vi "create.vi"(8 "error in (no error)":errorcluster, 11 "Type":T1=enum."FGEN_NI") -> (0 "error out":errorcluster, 3 "Fgen.lvclass":refnum<class "Arb.lvclass">)   [LabVIEW 2023, in "sweArb.lvlib" / "Arb.lvclass"]
doc: "<b>Author:</b> Wolfgang\n<b>Description:</b> Creates new Multimeter Object by type"
uses:
  Arb.lvclass
  Data/arbType.ctl
  sweArb.lvlib
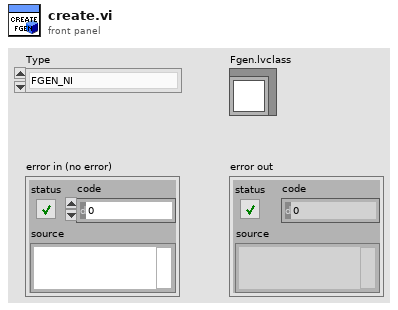
[diagram p1: front panel]
types:
  T1 = typedef "sweArb.lvlib/arbType.ctl" = enum16{"Simulated", "FGEN_NI", "FGEN_Keysight"}
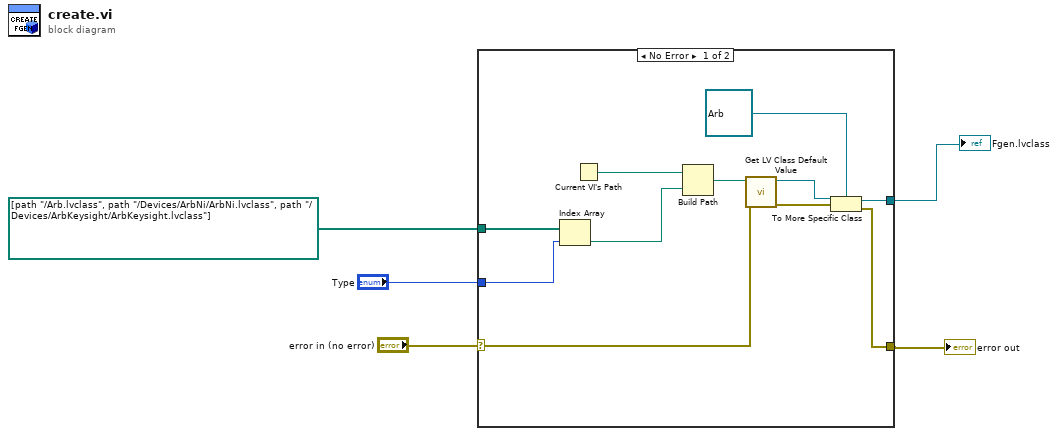
[diagram p0: block diagram]
diagram:
  n1 = case shown="No Error" "error in (no error)" {
    selector: "error in (no error)" -> [w15 w17]
    tunnel: [w13 _] -> w5
    tunnel: path[] [path "../Arb.lvclass", path "../Devices/ArbNi/ArbNi.lvclass", path "../Devices/ArbKeysight/ArbKeysight.lvclass"] ("Relative Paths") -> [w12 _]
    tunnel: "Type" -> [w10 _]
    tunnel: [w7 w17] -> w4
    frame No Error {
      n2 = Index Array(array=w12, index=w10) -> (element=w11:path)
      n3 = Current VI's Path() -> (path=w16:path)
      n4 = Build Path(base path=w16, name or relative path=w11) -> (appended path=w14:path)
      n5 = call <vilib>:"Get LV Class Default Value.vi"("error in (no error)"=w15, "class path"=w14) -> ("error out"=w9:errorcluster, "object"=w8:refnum<class>)  [unwired: 8 in]
      n6 = To More Specific Class(target class=refnum<class "Arb.lvclass"> refnum ("Fgen.lvclass"), reference=w8, error in=w9) -> (specific class reference=w13:refnum<class "Arb.lvclass">, error out=w7:errorcluster)
    }
    frame Error {
    }
  }
  "Fgen.lvclass" <- w5
  "error out" <- w4
